vi "Periodic Tasks.vi"(8 "error in":errorcluster) -> ()   [LabVIEW 2019]
doc: "This VI runs in parallel to other tasks. It can contain as many user-defined periodic loops as you need. These can carry out PID or other sorts of timed response."
uses:
  Robot Global Data.vi
  <vilib>/Rock Robotics/WPI/ThirdParty/Phoenix-LabVIEW/Motor Controller/Controls/CTRE_Phoenix_MotorControl_ControlMode.ctl
  <vilib>/addons/control/pid/NI_PID_pid.lvlib
  <vilib>/Rock Robotics/Network Tables/NT Write Number.vi
  <vilib>/Rock Robotics/WPI/ThirdParty/Phoenix-LabVIEW/Motor Controller/Get/CTRE_Phoenix_MotorController_GetQuadratureData.vi
  <vilib>/addons/control/pid/pid.llb/PID (DBL).vi
  servoCameraStates.ctl
  <vilib>/Rock Robotics/WPI/ThirdParty/Phoenix-LabVIEW/Motor Controller/Controls/CTRE_Phoenix_MotorControl_LimitSwitchSource_Local.ctl
  <vilib>/Rock Robotics/WPI/ThirdParty/Phoenix-LabVIEW/Motor Controller/Controls/CTRE_Phoenix_MotorControl_LimitSwitchNormal.ctl
  <vilib>/Rock Robotics/WPI/ThirdParty/Phoenix-LabVIEW/Motor Controller/Get/CTRE_Phoenix_MotorController_GetLimitSwitchStates.vi
  <vilib>/Rock Robotics/Network Tables/NT Read Number.vi
panel:
  out "Waveform Chart":T1(graph)
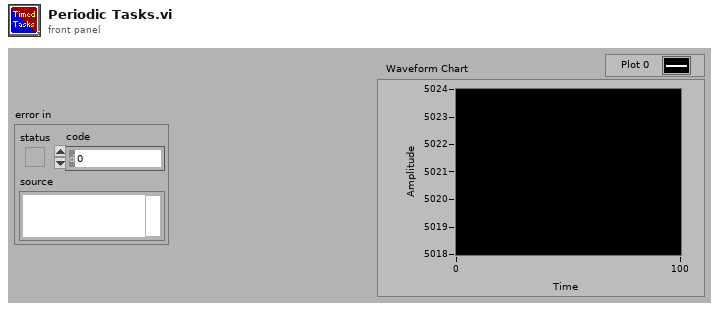
[diagram p1: front panel]
types:
  T1 = cluster{"intakePivotMotorActualAngle":dbl, "intakePivotMotorWantedAngle":dbl}
  T2 = typedef "CTRE_Phoenix_MotorControl_ControlMode.ctl" = u16
  T3 = typedef "WPI_MotorControlDeviceRef.ctl" = cluster{"DeviceStatus":errorcluster, "Type":T4, "PWM":cluster{"PWM Channel":T5, "DeadBand":T6}, "CAN":cluster{"Device Number":u8, "SetOutput VI Ref":variant, "GetOutput VI Ref":variant, "Enable VI Ref":variant, "Disable VI Ref":variant, "Data":variant}, "Invert":bool, "DIO PWM":cluster{"PWM \"Enable\" Channel":T5, "DIOChannel":T7, "PWM Rate":dbl}}
  T4 = typedef "WPI_MotorControlType.ctl" = enum16{"PWM", "CAN", "DIO PWM"}
  T5 = typedef "FPGA_DIOPWMChannel.ctl" = enum8{"PWM 0", "PWM 1", "PWM 2", "PWM 3", "PWM 4", "PWM 5", "PWM 6", "PWM 7", "PWM 8", "PWM 9", "PWM MXP 0", "PWM MXP 1", "PWM MXP 2", "PWM MXP 3", "PWM MXP 4", "PWM MXP 5", "PWM MXP 6", "PWM MXP 7", "PWM MXP 8", "PWM MXP 9", "Invalid"}
  T6 = typedef "WPI_PWMDeadband.ctl" = cluster{"Name":string, "maxPositivePwm":i32, "minPositivePwm":i32, "centerPwm":i32, "maxNegativePwm":i32, "minNegativePwm":i32, "angularRange":u16}
  T7 = typedef "FPGA_DIOChannel.ctl" = enum8{"DIO 0", "DIO 1", "DIO 2", "DIO 3", "DIO 4", "DIO 5", "DIO 6", "DIO 7", "DIO 8", "DIO 9", "DIO MXP 0", "DIO MXP 1", "DIO MXP 2", "DIO MXP 3", "DIO MXP 4", "DIO MXP 5", "DIO MXP 6", "DIO MXP 7", "DIO MXP 8", "DIO MXP 9", "DIO MXP 10", "DIO MXP 11", "DIO MXP 12", "DIO MXP 13", "DIO MXP 14", "DIO MXP 15", "SPI Port CS1", "SPI Port CS2", "SPI Port CS3", "SPI Port MISO", "SPI Port MOSI", "Invalid"}
  T8 = typedef "WPI_DriverStationRobotMode2.ctl" = enum16{"Autonomous Disabled", "Autonomous Enabled", "Teleop Disabled", "Teleop Enabled", "Disconnected", "Finish", "Test Disabled", "Test Enabled", "Emergency Stopped"}
  T9 = typedef "WPI_RobotDriveDevRef.ctl" = cluster{"DevStatus":errorcluster, "Motors[]":T3[], "Square Inputs":bool, "Max Output":dbl}
  T10 = cluster{"proportional gain (Kc)":dbl, "integral time (Ti, min)":dbl, "derivative time (Td, min)":dbl}
  T11 = typedef "CTRE_Phoenix_MotorControl_LimitSwitchNormal.ctl" = enum16{"Normally Open", "Normally Closed", "Disabled"}
  T12 = typedef "CTRE_Phoenix_MotorControl_LimitSwitchSource_Local.ctl" = enum16{"Feedback Connector", "Remote Talon SRX", "Remote CANifier", "Deactivated"}
  T13 = typedef "servoCameraStates.ctl" = enum16{"Up", "Out", "Down", ""}
  T14 = typedef "WPI_ServoDeviceRef.ctl" = cluster{"DeviceStatus":errorcluster, "PWM Channel":T5, "DeadBand":T6}
  T15 = typedef "WPI_CounterDevRef.ctl" = cluster{"DevStatus":errorcluster, "CntIndex":T16}
  T16 = typedef "FPGA_CounterCtrSystemIndex.ctl" = enum8{"Ctr 0", "Ctr 1", "Ctr 2", "Ctr 3", "Ctr 4", "Ctr 5", "Ctr 6", "Ctr 7", "Invalid"}
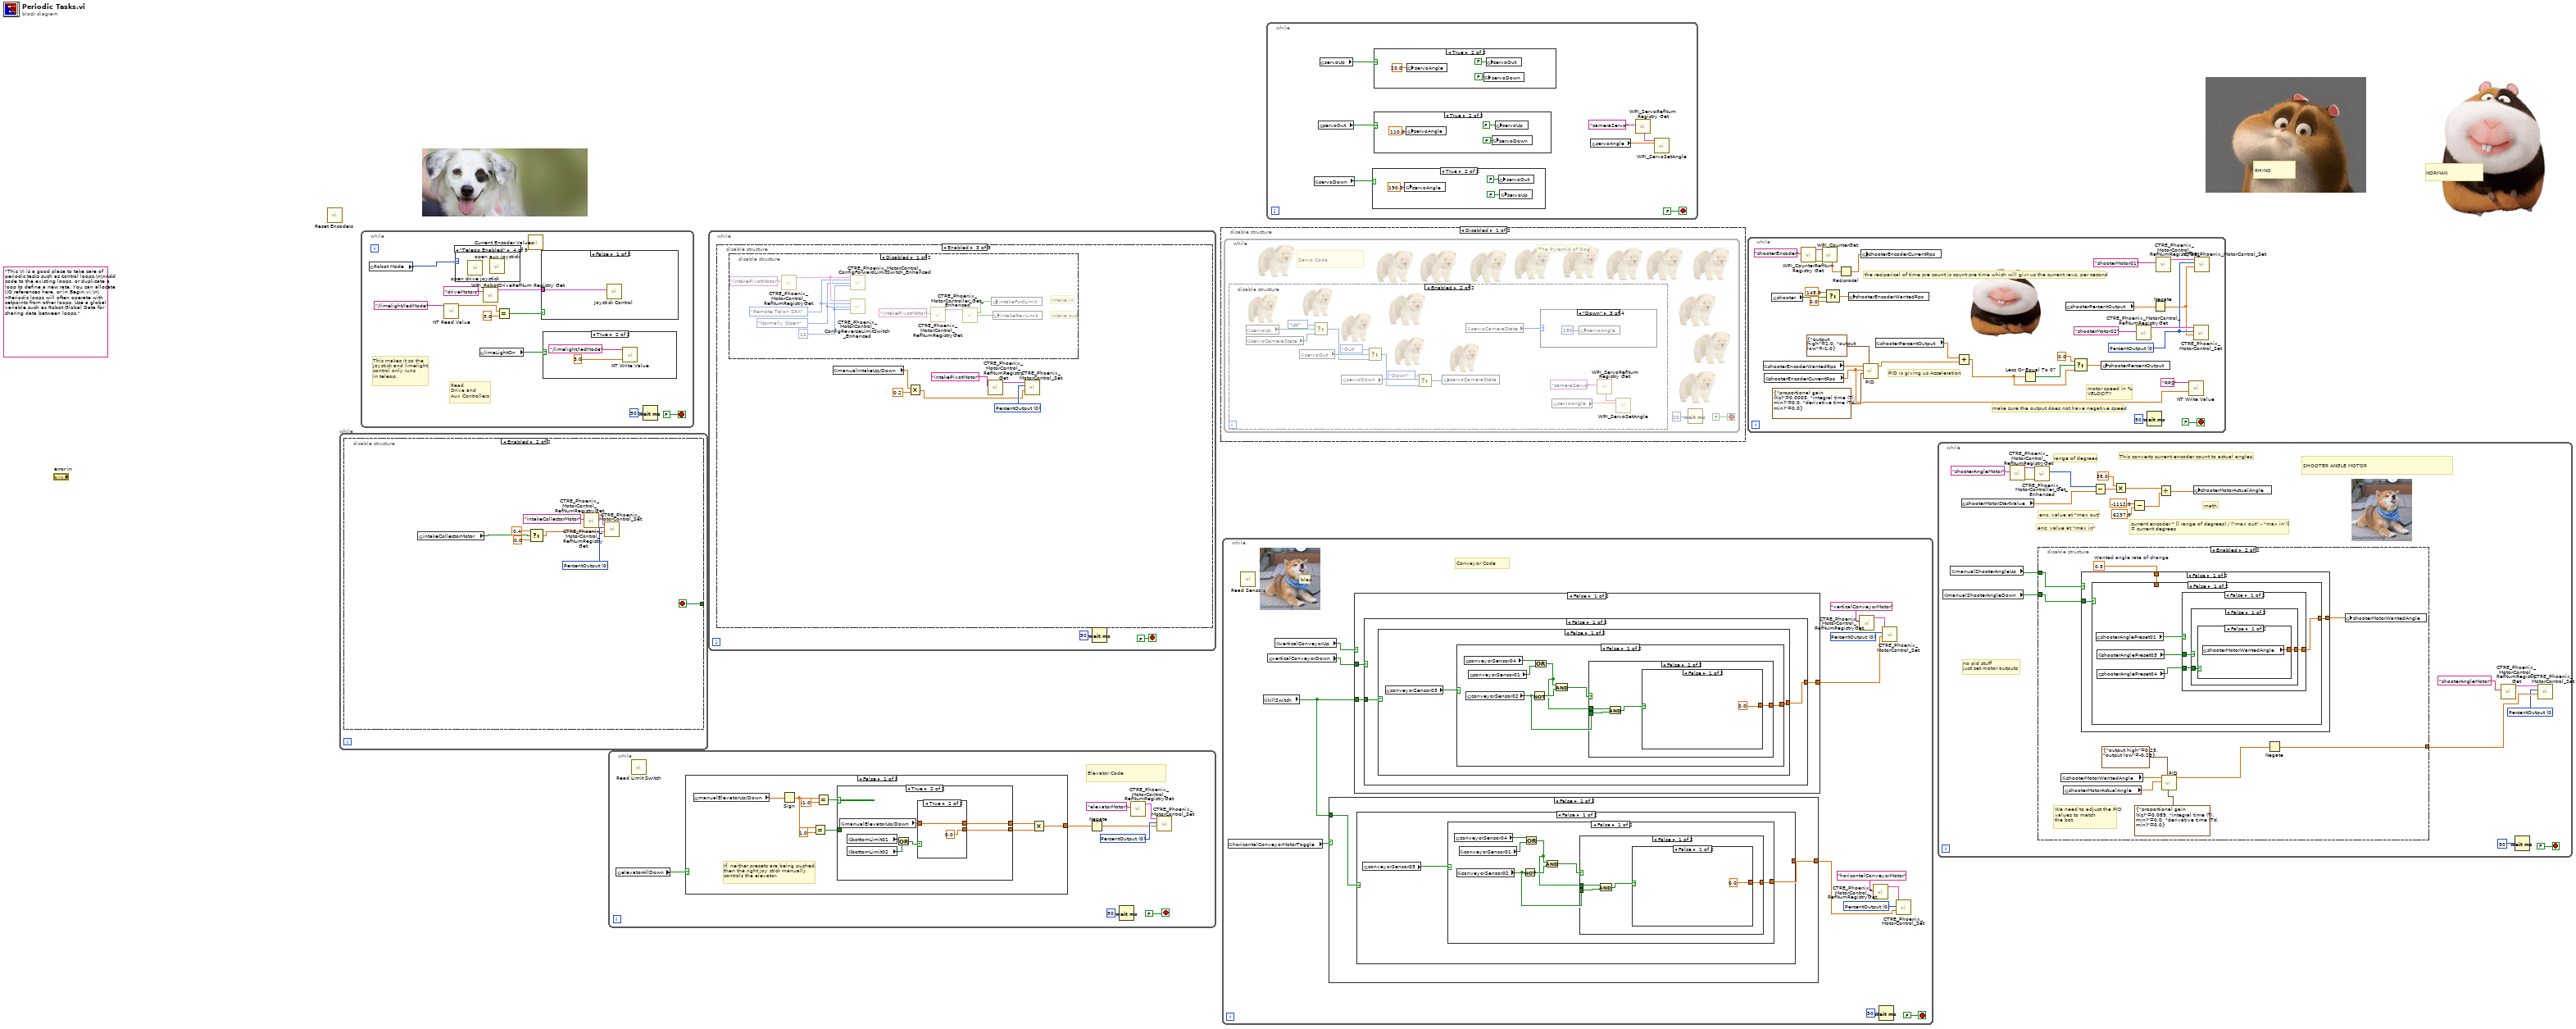
[diagram p0: block diagram]
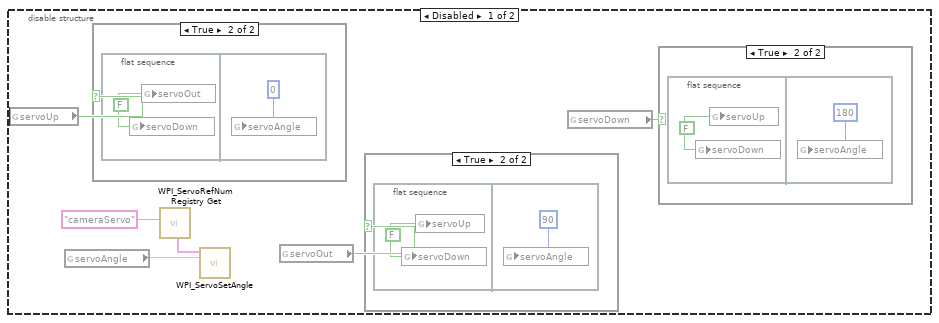
[diagram p5: hidden frame]
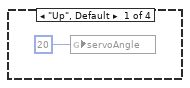
[diagram p9: hidden frame]
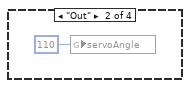
[diagram p10: hidden frame]
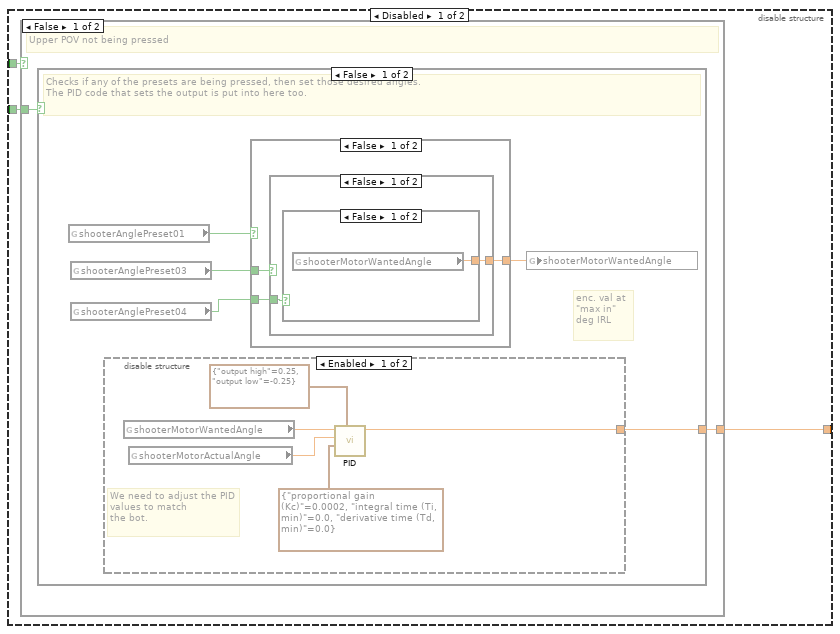
[diagram p13: hidden frame]
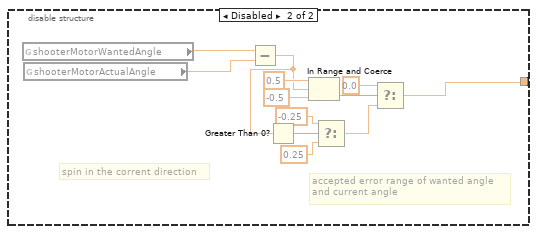
[diagram p14: hidden frame]
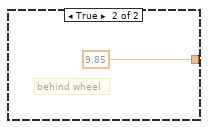
[diagram p15: hidden frame]
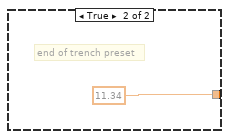
[diagram p16: hidden frame]
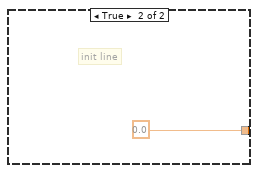
[diagram p17: hidden frame]
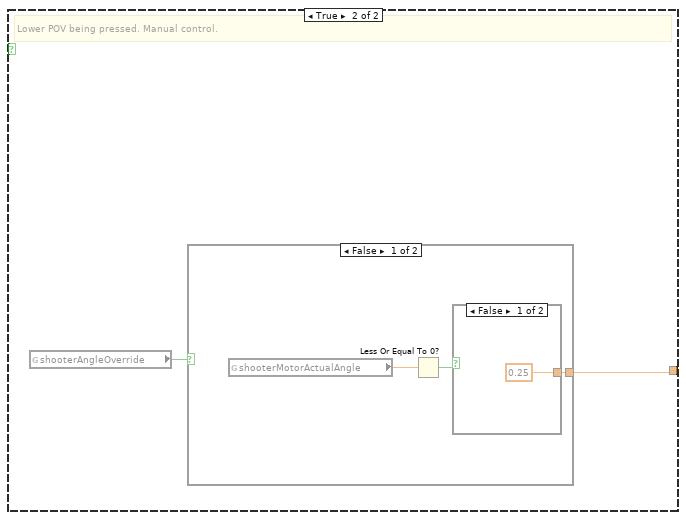
[diagram p18: hidden frame]
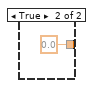
[diagram p19: hidden frame]
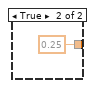
[diagram p20: hidden frame]
diagram:
  (unwired) "This VI is a good place to take care of periodic tasks such as control loops.\n\nAdd code to the existing loops, or duplicate a loop to define a new rate. You can allocate I/O references here, or in Begin.vi.\n\nPeriodic loops will often operate with setpoints from other loops. Use a global variable such as Robot Global Data for sharing data between loops."
  # "RHINO"
  # "NORMAN"
  n1 = call "Reset Encoders.vi"() -> ()  [unwired: 12 in]
  n2 = while {
    stop <- w1 stop-if-true
    n3 = disable-structure shown="Enabled" {
      disable-tunnel: [FALSE _] -> w1
      frame Disabled {
        w17 = T2 0 items=["PercentOutput"=0, "Position"=1, "Velocity"=2, "Current"=3, "Follower"=5, "MotionProfile"=6, "MotionMagic"=7, "MotionProfileArc"=10, "Disabled"=15] ("Control Mode")
        # "math"
        # "current encoder * [( range of degrees) / (\"max out\" - \"max in')]\n= current degrees"
        # "enc. value at \"max in\""
        # "enc. value at \"max out\""
        # "This converts current encoder count to actual angles."
        # "range of degrees"
        # "Check if motor value\nneeds to be negative\nor not."
        # "This chunk of code checks the current angle of the \nintake pivot motor. \nIf the motor is at or more of the desired \"all the way out\" \nangle then the intake collector motor begins to spin.\nIf the angle goes out of the range the motor will stop."
        # "All the way out intake angle."
        # "Intake Collector Code"
        n4 = global read "Robot Global Data.vi" "intakePivotMotorStartValue"() -> (w10:dbl)
        n5 = call <vilib>:"CTRE_Phoenix_MotorControl_RefNumRegistryGet.vi"("refnum name"="intakePivotMotor") -> ("error out"=w11:errorcluster, "PhoenixMotorControlDevRef"=w12:T3)  [unwired: 9 in]
        n6 = call-poly <vilib>:"CTRE_Phoenix_MotorController_Get_Enhanced.vi"("PhoenixMotorControlDevRef"=w12, "error in"=w11) -> ("Quadrature Position"=w2:i32)  [unwired: 10 in, 3 out]
        n7 = global read "Robot Global Data.vi" "intakePivotMotorActualAngle"() -> (w21:dbl)
        n8 = global write "Robot Global Data.vi" "intakePivotMotorActualValue"(w2) -> ()
        n9 = Subtract(x=w2, y=w10) -> (x-y=w9:dbl)
        n10 = Greater Or Equal?(x=w21, y=35.0 ("upper limit")) -> (x >= y?=w19:bool)
        n11 = Multiply(x=87.0, y=w9) -> (x*y=w5:dbl)
        n12 = case shown="True" w19 {
          tunnel: [0.0 0.4] -> w15
          frame False {
          }
          frame True {
          }
        }
        n13 = Subtract(x=-851.0, y=-20.0) -> (x-y=w4:dbl)
        n14 = Divide(x=w5, y=w4) -> (x/y=w3:dbl)
        n15 = global write "Robot Global Data.vi" "intakePivotMotorActualAngle"(w3) -> ()
        n16 = Wait (ms)(milliseconds to wait=u32 50) -> ()  [unwired: 1 out]
        n17 = call <vilib>:"CTRE_Phoenix_MotorControl_RefNumRegistryGet.vi"("refnum name"="intakeCollectorMotor") -> ("PhoenixMotorControlDevRef"=w18:T3)  [unwired: 9 in, 1 out]
        n18 = call <vilib>:"CTRE_Phoenix_MotorControl_Set.vi"("Output"=w15, "Control Mode"=w17, "PhoenixMotorControlDevRef"=w18) -> ()  [unwired: 7 in, 2 out]
      }
      frame Enabled {
        w30 = T2 0 items=["PercentOutput"=0, "Position"=1, "Velocity"=2, "Current"=3, "Follower"=5, "MotionProfile"=6, "MotionMagic"=7, "MotionProfileArc"=10, "Disabled"=15] ("Control Mode")
        (unwired) T2 0 items=["PercentOutput"=0, "Position"=1, "Velocity"=2, "Current"=3, "Follower"=5, "MotionProfile"=6, "MotionMagic"=7, "MotionProfileArc"=10, "Disabled"=15] ("Control Mode")
        n19 = global read "Robot Global Data.vi" "intakeCollectorMotor"() -> (w25:bool)
        n20 = Select(t=0.4, s=w25, f=0.0) -> (s? t:f=w28:dbl)
        n21 = call <vilib>:"CTRE_Phoenix_MotorControl_RefNumRegistryGet.vi"("refnum name"="intakeCollectorMotor") -> ("PhoenixMotorControlDevRef"=w31:T3)  [unwired: 9 in, 1 out]
        n22 = call <vilib>:"CTRE_Phoenix_MotorControl_RefNumRegistryGet.vi"("refnum name"="intakeCollectorMotor") -> ()  [unwired: 9 in, 2 out]
        n23 = call <vilib>:"CTRE_Phoenix_MotorControl_Set.vi"("Output"=w28, "Control Mode"=w30, "PhoenixMotorControlDevRef"=w31) -> ()  [unwired: 7 in, 2 out]
      }
    }
  }
  n24 = while {
    stop <- FALSE stop-if-true
    # "Read\nDrive and\nAux Controllers"
    # "This makes it so the\njoystick and limelight\ncontrol only runs\nin teleop."
    n25 = global read "Robot Global Data.vi" "Robot Mode"() -> (w33:T8)
    n26 = call-poly <vilib>:"NT Read Value.vi"("Name"="/limelight/ledMode") -> ("Numeric"=w35:dbl)  [unwired: 9 in, 1 out]
    n27 = case shown="\"Teleop Enabled\"" w33 {
      frame "Autonomous Disabled", Default {
        n28 = call "open drive joystick.vi"() -> ()  [unwired: 12 in]
        n29 = call "open aux joystick.vi"() -> ()  [unwired: 12 in]
      }
      frame "Autonomous Enabled" {
      }
      frame "Teleop Disabled" {
        n30 = call "open drive joystick.vi"() -> ()  [unwired: 12 in]
        n31 = call "open aux joystick.vi"() -> ()  [unwired: 12 in]
      }
      frame "Teleop Enabled" {
        n32 = call "open drive joystick.vi"() -> ()  [unwired: 12 in]
        n33 = call "open aux joystick.vi"() -> ()  [unwired: 12 in]
      }
      frame "Disconnected" {
        n34 = call "open drive joystick.vi"() -> ()  [unwired: 12 in]
        n35 = call "open aux joystick.vi"() -> ()  [unwired: 12 in]
      }
      frame "Finish" {
        n36 = call "open drive joystick.vi"() -> ()  [unwired: 12 in]
        n37 = call "open aux joystick.vi"() -> ()  [unwired: 12 in]
      }
      frame "Test Disabled" {
        n38 = call "open drive joystick.vi"() -> ()  [unwired: 12 in]
        n39 = call "open aux joystick.vi"() -> ()  [unwired: 12 in]
      }
      frame "Test Enabled" {
        n40 = call "open drive joystick.vi"() -> ()  [unwired: 12 in]
        n41 = call "open aux joystick.vi"() -> ()  [unwired: 12 in]
      }
      frame "Emergency Stopped" {
        n42 = call "open drive joystick.vi"() -> ()  [unwired: 12 in]
        n43 = call "open aux joystick.vi"() -> ()  [unwired: 12 in]
      }
    }
    n44 = global read "Robot Global Data.vi" "limeLightOn"() -> (w38:bool)
    n45 = call <vilib>:"WPI_RobotDriveRefNum Registry Get.vi"("refnum name"="driveMotors") -> ("RobotDriveDevRef"=w39:T9)  [unwired: 9 in, 1 out]
    n46 = Equal?(x=w35, y=3.0) -> (x = y?=w34:bool)
    n47 = call "Current Encoder Values.vi"() -> ()  [unwired: 12 in]
    n48 = case shown="False" w34 {
      tunnel: w39 -> [w47 w48]
      frame False {
        n49 = call "Joystick Control.vi"("RobotDriveDevRef"=w47) -> ()  [unwired: 11 in]
      }
      frame True {
        # "sounds cool"
        n50 = call "Limelight Control.vi"("input cluster"=w48) -> ()  [unwired: 11 in]
      }
    }
    n51 = case shown="True" w38 {
      frame False {
        n52 = call-poly <vilib>:"NT Write Value.vi"("Numeric"=1.0, "Name"="/limelight/ledMode") -> ()  [unwired: 9 in, 1 out]
      }
      frame True {
        n53 = call-poly <vilib>:"NT Write Value.vi"("Numeric"=3.0, "Name"="/limelight/ledMode") -> ()  [unwired: 9 in, 1 out]
      }
    }
    n54 = Wait (ms)(milliseconds to wait=u32 50) -> ()  [unwired: 1 out]
  }
  n55 = while {
    stop <- FALSE stop-if-true
    w53 = T2 0 items=["PercentOutput"=0, "Position"=1, "Velocity"=2, "Current"=3, "Follower"=5, "MotionProfile"=6, "MotionMagic"=7, "MotionProfileArc"=10, "Disabled"=15] ("Control Mode")
    # "Elevator Code"
    n56 = global read "Robot Global Data.vi" "elevatorAllDown"() -> (w50:bool)
    n57 = call "Read Limit Switch.vi"() -> ()  [unwired: 12 in]
    n58 = case shown="False" w50 {
      tunnel: [w65 w94] -> w51
      frame False {
        # "If, neither presets are being pushed, \nthen the right joy stick manually \ncontrols the elevator."
        n59 = global read "Robot Global Data.vi" "manualElevatorUp/Down"() -> (w64:dbl)
        n60 = Sign(1:w64) -> (0:w59:dbl)
        n61 = Equal?(x=w59, y=1.0) -> (x = y?=w57:bool)
        n62 = Equal?(x=w59, y=-1.0) -> (x = y?=w63:bool)
        n63 = case shown="True" w63 {
          tunnel: [w66 w83] -> w61
          tunnel: [w67 w81] -> w60
          tunnel: w57 -> [w68 _]
          frame False {
            n64 = case shown="False" w68 {
              tunnel: [0.0 w73] -> w67
              tunnel: [0.0 w72] -> w66
              frame False {
              }
              frame True {
                n65 = global read "Robot Global Data.vi" "manualElevatorUp/Down"() -> (w74:dbl)
                n66 = global read "Robot Global Data.vi" "upperLimit01"() -> (w75:bool)
                n67 = global read "Robot Global Data.vi" "upperLimit02"() -> (w76:bool)
                n68 = Or(x=w75, y=w76) -> (x .or. y?=w71:bool)
                n69 = case shown="False" w71 {
                  tunnel: w74 -> [w77 w80]
                  tunnel: [w77 w80] -> w73
                  tunnel: [1.0 0.0] -> w72
                  frame False {
                  }
                  frame True {
                  }
                }
              }
            }
          }
          frame True {
            n70 = global read "Robot Global Data.vi" "manualElevatorUp/Down"() -> (w82:dbl)
            n71 = global read "Robot Global Data.vi" "bottomLimit01"() -> (w85:bool)
            n72 = global read "Robot Global Data.vi" "bottomLimit02"() -> (w86:bool)
            n73 = Or(x=w85, y=w86) -> (x .or. y?=w84:bool)
            n74 = case shown="True" w84 {
              tunnel: [1.0 0.0] -> w83
              tunnel: w82 -> [w88 w89]
              tunnel: [w88 w89] -> w81
              frame False {
              }
              frame True {
              }
            }
          }
        }
        n75 = Multiply(x=w60, y=w61) -> (x*y=w65:dbl)
      }
      frame True {
        # "the elevator will keep moving down\nuntil the lower limit switch turns true."
        n76 = global read "Robot Global Data.vi" "bottomLimit01"() -> (w91:bool)
        n77 = global read "Robot Global Data.vi" "bottomLimit02"() -> (w92:bool)
        n78 = Or(x=w91, y=w92) -> (x .or. y?=w93:bool)
        n79 = case shown="False" w93 {
          tunnel: [w95 0.0] -> w94
          frame False {
            n80 = Negate(x=0.8) -> (-x=w95:dbl)
          }
          frame True {
          }
        }
      }
    }
    n81 = Negate(x=w51) -> (-x=w49:dbl)
    n82 = Wait (ms)(milliseconds to wait=u32 50) -> ()  [unwired: 1 out]
    n83 = call <vilib>:"CTRE_Phoenix_MotorControl_RefNumRegistryGet.vi"("refnum name"="elevatorMotor") -> ("PhoenixMotorControlDevRef"=w52:T3)  [unwired: 9 in, 1 out]
    n84 = call <vilib>:"CTRE_Phoenix_MotorControl_Set.vi"("Output"=w49, "Control Mode"=w53, "PhoenixMotorControlDevRef"=w52) -> ()  [unwired: 7 in, 2 out]
  }
  n85 = while {
    stop <- FALSE stop-if-true
    n86 = disable-structure shown="Enabled" {
      frame Disabled {
        w116 = T2 0 items=["PercentOutput"=0, "Position"=1, "Velocity"=2, "Current"=3, "Follower"=5, "MotionProfile"=6, "MotionMagic"=7, "MotionProfileArc"=10, "Disabled"=15] ("Control Mode")
        # "This chunk of code actually gives the\nintake pivot motor a value by comparing\nthe actual to the wanted and then doing \nmath."
        # "This chunk of code see's if either preset\nbutton is being pressed, then gives the\ndesired angle depending on which button\nis being pressed. If neither button is being\npressed, then the left joystick on the aux\ncontrols the pivot motor."
        # "We need to adjust the PID values to match \nthe bot."
        # "We need to get the preset\nangles for the intake as \nsoon as we get the robot."
        # "Use this to scale the rate at which the\nwanted angle changes based on the joystick"
        n87 = global read "Robot Global Data.vi" "intakePivotMotorWantedAngle"() -> (w103:dbl)
        n88 = global read "Robot Global Data.vi" "intakePivotMotorActualAngle"() -> (w104:dbl)
        n89 = global read "Robot Global Data.vi" "manualIntakeUp/Down"() -> (w125:dbl)
        n90 = global read "Robot Global Data.vi" "intakeOut"() -> (w124:bool)
        n91 = global read "Robot Global Data.vi" "intakeIn"() -> (w122)
        n92 = Or(x=w122, y=w124) -> (x .or. y?=w123:bool)
        n93 = call <vilib>:"CTRE_Phoenix_MotorControl_RefNumRegistryGet.vi"("refnum name"="intakePivotMotor") -> ("error out"=w113:errorcluster, "PhoenixMotorControlDevRef"=w114:T3)  [unwired: 9 in]
        n94 = Multiply(x=1.0, y=w125) -> (x*y=w120:dbl)
        n95 = call-poly <vilib>:"CTRE_Phoenix_MotorController_Get_Enhanced.vi"("PhoenixMotorControlDevRef"=w114, "error in"=w113) -> ("Quadrature Position"=w111:i32)  [unwired: 10 in, 3 out]
        n96 = call-poly <vilib>:"PID.vi"("output range"=cluster{"output high":dbl, "output low":dbl} {"output high"=0.2, "output low"=-0.2}, "PID gains"=T10 {"proportional gain (Kc)"=0.015, "integral time (Ti, min)"=0.0, "derivative time (Td, min)"=0.0}, "process variable"=w103, "setpoint"=w104) -> ("output"=w101:dbl)  [unwired: 6 in, 1 out]
        n97 = case shown="False" w123 {
          tunnel: w122 -> [_ w131]
          tunnel: [w127 w130] -> w121
          tunnel: w120 -> [w128 _]
          frame False {
            # "Neither Preset buttons \nare being pressed.\n\nThis allows the Left Y\njoystick to control the \nActual Angle"
            n98 = global read "Robot Global Data.vi" "intakePivotMotorWantedAngle"() -> (w129:dbl)
            n99 = Add(x=w129, y=w128) -> (x+y=w127:dbl)
          }
          frame True {
            n100 = case shown="False" w131 {
              tunnel: [5018.0 5192.0] -> w130
              frame False {
                # "Preset angle for \nintake at Out Position"
              }
              frame True {
                # "Preset Angle for\nIntake at Vertical \nPosition"
              }
            }
          }
        }
        n101 = Negate(x=w101) -> (-x=w100:dbl)
        n102 = Subtract(x=960.0, y=24.0) -> (x-y=w107:dbl)
        n103 = Bundle("intakePivotMotorActualAngle"=w104, "intakePivotMotorWantedAngle"=w103) -> (→"Waveform Chart":T1)  [unwired: 1 in]
        n104 = call <vilib>:"CTRE_Phoenix_MotorControl_RefNumRegistryGet.vi"("refnum name"="intakePivotMotor") -> ("PhoenixMotorControlDevRef"=w117:T3)  [unwired: 9 in, 1 out]
        n105 = Divide(x=180.0, y=w107) -> (x/y=w106:dbl)
        n106 = call <vilib>:"CTRE_Phoenix_MotorControl_Set.vi"("Output"=w100, "Control Mode"=w116, "PhoenixMotorControlDevRef"=w117) -> ()  [unwired: 7 in, 2 out]
        n107 = Multiply(x=w106, y=w111) -> (x*y=w112:dbl)
        n108 = global write "Robot Global Data.vi" "intakePivotMotorActualAngle"(w112) -> ()
        n109 = global write "Robot Global Data.vi" "intakePivotMotorWantedAngle"(w121) -> ()
      }
      frame Disabled {
        w149 = T2 0 items=["PercentOutput"=0, "Position"=1, "Velocity"=2, "Current"=3, "Follower"=5, "MotionProfile"=6, "MotionMagic"=7, "MotionProfileArc"=10, "Disabled"=15] ("Control Mode")
        # "INTAKE PIVOT MOTOR CODE"
        # "math"
        # "current encoder * [( range of degrees) / (\"max out\" - \"max in')]\n= current degrees"
        # "enc. value at \"max in\""
        # "enc. value at \"max out\""
        # "This converts current encoder count to actual angles."
        # "range of degrees"
        n110 = global read "Robot Global Data.vi" "intakePivotMotorStartValue"() -> (w142:dbl)
        n111 = call <vilib>:"CTRE_Phoenix_MotorControl_RefNumRegistryGet.vi"("refnum name"="intakePivotMotor") -> ("error out"=w143:errorcluster, "PhoenixMotorControlDevRef"=w144:T3)  [unwired: 9 in]
        n112 = global read "Robot Global Data.vi" "manualIntakeUp/Down"() -> (w148:dbl)
        n113 = call-poly <vilib>:"CTRE_Phoenix_MotorController_Get_Enhanced.vi"("PhoenixMotorControlDevRef"=w144, "error in"=w143) -> ("Quadrature Position"=w134:i32)  [unwired: 10 in, 3 out]
        n114 = global write "Robot Global Data.vi" "intakePivotMotorActualValue"(w134) -> ()
        n115 = Multiply(x=w148, y=0.2) -> (x*y=w146:dbl)
        n116 = Subtract(x=w134, y=w142) -> (x-y=w141:dbl)
        n117 = Multiply(x=87.0, y=w141) -> (x*y=w137:dbl)
        n118 = Subtract(x=-851.0, y=-20.0) -> (x-y=w136:dbl)
        n119 = call <vilib>:"CTRE_Phoenix_MotorControl_RefNumRegistryGet.vi"("refnum name"="intakePivotMotor") -> ("PhoenixMotorControlDevRef"=w150:T3)  [unwired: 9 in, 1 out]
        n120 = Divide(x=w137, y=w136) -> (x/y=w135:dbl)
        n121 = call <vilib>:"CTRE_Phoenix_MotorControl_Set.vi"("Output"=w146, "Control Mode"=w149, "PhoenixMotorControlDevRef"=w150) -> ()  [unwired: 7 in, 2 out]
        n122 = global write "Robot Global Data.vi" "intakePivotMotorActualAngle"(w135) -> ()
      }
      frame Enabled {
        w155 = T2 0 items=["PercentOutput"=0, "Position"=1, "Velocity"=2, "Current"=3, "Follower"=5, "MotionProfile"=6, "MotionMagic"=7, "MotionProfileArc"=10, "Disabled"=15] ("Control Mode")
        n123 = disable-structure shown="Disabled" {
          frame Disabled {
            w164 = 10 ("deviceID")
            w163 = CTRE_Phoenix_MotorControl_LimitSwitchNormal."Normally Open" ("NormallyOpenOrClosed")
            w162 = CTRE_Phoenix_MotorControl_LimitSwitchSource_Local."Remote Talon SRX" ("Limit Switch Source")
            # "intake out"
            # "intake in"
            n124 = call <vilib>:"CTRE_Phoenix_MotorControl_RefNumRegistryGet.vi"("refnum name"="intakePivotMotor") -> ("PhoenixMotorControlDevRef"=w165:T3)  [unwired: 9 in, 1 out]
            n125 = call <vilib>:"CTRE_Phoenix_MotorControl_ConfigForwardLimitSwitch_Enhanced.vi"("PhoenixMotorControlDevRef"=w165, "Limit Switch Source"=w162, "NormallyOpenOrClosed"=w163, "deviceID"=w164) -> ()  [unwired: 10 in, 2 out]
            n126 = call <vilib>:"CTRE_Phoenix_MotorControl_ConfigReverseLimitSwitch_Enhanced.vi"("PhoenixMotorControlDevRef"=w165, "Limit Switch Source"=w162, "NormallyOpenOrClosed"=w163, "deviceID"=w164) -> ()  [unwired: 10 in, 2 out]
            n127 = call <vilib>:"CTRE_Phoenix_MotorControl_RefNumRegistryGet.vi"("refnum name"="intakePivotMotor") -> ("PhoenixMotorControlDevRef"=w161:T3)  [unwired: 9 in, 1 out]
            n128 = call-poly <vilib>:"CTRE_Phoenix_MotorController_Get_Enhanced.vi"("PhoenixMotorControlDevRef"=w161) -> ("Forward Limit Closed?"=w158:bool, "Reverse Limit Closed?"=w159:bool)  [unwired: 11 in, 2 out]
            n129 = global write "Robot Global Data.vi" "intakeFwdLimit"(w158) -> ()
            n130 = global write "Robot Global Data.vi" "intakeRevLimit"(w159) -> ()
          }
          frame Enabled {
          }
        }
        n131 = global read "Robot Global Data.vi" "manualIntakeUp/Down"() -> (w154:dbl)
        n132 = Multiply(x=w154, y=0.2) -> (x*y=w152:dbl)
        n133 = call <vilib>:"CTRE_Phoenix_MotorControl_RefNumRegistryGet.vi"("refnum name"="intakePivotMotor") -> ("PhoenixMotorControlDevRef"=w156:T3)  [unwired: 9 in, 1 out]
        n134 = call <vilib>:"CTRE_Phoenix_MotorControl_Set.vi"("Output"=w152, "Control Mode"=w155, "PhoenixMotorControlDevRef"=w156) -> ()  [unwired: 7 in, 2 out]
      }
      frame Disabled {
        w169 = T2 0 items=["PercentOutput"=0, "Position"=1, "Velocity"=2, "Current"=3, "Follower"=5, "MotionProfile"=6, "MotionMagic"=7, "MotionProfileArc"=10, "Disabled"=15] ("Control Mode")
        n135 = global read "Robot Global Data.vi" "manualIntakeUp/Down"() -> (w167:dbl)
        n136 = global read "Robot Global Data.vi" "intakeOut"() -> (w176:bool)
        n137 = global read "Robot Global Data.vi" "intakeIn"() -> (w178)
        n138 = Or(x=w178, y=w176) -> (x .or. y?=w177:bool)
        n139 = call <vilib>:"CTRE_Phoenix_MotorControl_RefNumRegistryGet.vi"("refnum name"="intakePivotMotor") -> ("error out"=w180:errorcluster, "PhoenixMotorControlDevRef"=w179:T3)  [unwired: 9 in]
        n140 = call-poly <vilib>:"CTRE_Phoenix_MotorController_Get_Enhanced.vi"("PhoenixMotorControlDevRef"=w179, "error in"=w180) -> ("Quadrature Position"=w182:i32)  [unwired: 10 in, 3 out]
        n141 = case shown="False" w177 {
          tunnel: w178 -> [_ w189]
          tunnel: [w185 w188] -> w168
          tunnel: w167 -> [w186 _]
          frame False {
            # "Neither Preset buttons \nare being pressed.\n\nThis allows the Left Y\njoystick to control the \nActual Angle"
            n142 = Multiply(x=w186, y=0.2) -> (x*y=w185:dbl)
          }
          frame True {
            n143 = case shown="True" w189 {
              tunnel: [w193 w199] -> w188
              frame False {
                n144 = global read "Robot Global Data.vi" "intakePivotMotorActualAngle"() -> (w192:dbl)
                n145 = Less Or Equal?(x=w192, y=5018.0) -> (x <= y?=w190:bool)
                n146 = Select(t=0.0, s=w190, f=-0.2) -> (s? t:f=w193:dbl)
              }
              frame True {
                n147 = global read "Robot Global Data.vi" "intakePivotMotorActualAngle"() -> (w198:dbl)
                n148 = Greater Or Equal?(x=w198, y=5192.0) -> (x >= y?=w196:bool)
                n149 = Select(t=0.0, s=w196, f=0.2) -> (s? t:f=w199:dbl)
              }
            }
          }
        }
        n150 = Subtract(x=960.0, y=24.0) -> (x-y=w183:dbl)
        n151 = Divide(x=180.0, y=w183) -> (x/y=w184:dbl)
        n152 = Multiply(x=w184, y=w182) -> (x*y=w181:dbl)
        n153 = global write "Robot Global Data.vi" "intakePivotMotorActualAngle"(w181) -> ()
        n154 = call <vilib>:"CTRE_Phoenix_MotorControl_RefNumRegistryGet.vi"("refnum name"="intakePivotMotor") -> ("PhoenixMotorControlDevRef"=w170:T3)  [unwired: 9 in, 1 out]
        n155 = call <vilib>:"CTRE_Phoenix_MotorControl_Set.vi"("Output"=w168, "Control Mode"=w169, "PhoenixMotorControlDevRef"=w170) -> ()  [unwired: 7 in, 2 out]
      }
      frame Disabled {
        w218 = T2 0 items=["PercentOutput"=0, "Position"=1, "Velocity"=2, "Current"=3, "Follower"=5, "MotionProfile"=6, "MotionMagic"=7, "MotionProfileArc"=10, "Disabled"=15] ("Control Mode")
        # "0.017"
        # "prevent manuall adjustment from going out of\nacceptable angels. alos give the drivers the option to push\nfutther than the angel presets by 5 degrees."
        # "INTAKE PIVOT MOTOR CODE"
        # "We need to adjust the PID values to match \nthe bot."
        # "math"
        # "current encoder * [( range of degrees) / (\"max out\" - \"max in')]\n= current degrees"
        # "enc. value at \"max in\""
        # "enc. value at \"max out\""
        # "This converts current encoder count to actual angles."
        # "range of degrees"
        n156 = global read "Robot Global Data.vi" "manualIntakeUp/Down"() -> (w210:dbl)
        n157 = global read "Robot Global Data.vi" "intakePivotMotorStartValue"() -> (w232:dbl)
        n158 = global read "Robot Global Data.vi" "intakeOut"() -> (w216:bool)
        n159 = global read "Robot Global Data.vi" "intakeEat"() -> (w217:bool)
        n160 = global read "Robot Global Data.vi" "intakePivotMotorWantedAngle"() -> (w222:dbl)
        n161 = global read "Robot Global Data.vi" "intakePivotMotorActualAngle"() -> (w206:dbl)
        n162 = call <vilib>:"CTRE_Phoenix_MotorControl_RefNumRegistryGet.vi"("refnum name"="intakePivotMotor") -> ("error out"=w233:errorcluster, "PhoenixMotorControlDevRef"=w234:T3)  [unwired: 9 in]
        n163 = Negate(x=w210) -> (-x=w209:dbl)
        n164 = case shown="False" w217 {
          tunnel: w216 -> [w238 _]
          tunnel: [w237 -5.0] -> w214
          tunnel: w209 -> [w236 _]
          frame False {
            n165 = case shown="True" w238 {
              tunnel: [w239 85.0] -> w237
              tunnel: w236 -> [w242 _]
              frame False {
                # "Use this to scale the rate at which the\nwanted angle changes based on the joystick"
                n166 = global read "Robot Global Data.vi" "intakePivotMotorWantedAngle"() -> (w243:dbl)
                n167 = Multiply(x=w242, y=3.0) -> (x*y=w240:dbl)
                n168 = Add(x=w243, y=w240) -> (x+y=w239:dbl)
              }
              frame True {
              }
            }
          }
          frame True {
          }
        }
        n169 = call-poly <vilib>:"CTRE_Phoenix_MotorController_Get_Enhanced.vi"("PhoenixMotorControlDevRef"=w234, "error in"=w233) -> ("Quadrature Position"=w224:i32)  [unwired: 10 in, 3 out]
        n170 = global write "Robot Global Data.vi" "intakePivotMotorActualValue"(w224) -> ()
        n171 = call-poly <vilib>:"PID.vi"("output range"=cluster{"output high":dbl, "output low":dbl} {"output high"=0.2, "output low"=-0.2}, "PID gains"=T10 {"proportional gain (Kc)"=0.017, "integral time (Ti, min)"=0.0, "derivative time (Td, min)"=0.0}, "process variable"=w206, "setpoint"=w222) -> ("output"=w207:dbl)  [unwired: 6 in, 1 out]
        n172 = Subtract(x=w224, y=w232) -> (x-y=w231:dbl)
        n173 = Multiply(x=87.0, y=w231) -> (x*y=w227:dbl)
        n174 = Less Or Equal?(x=w206, y=45.0 ("x")) -> (x <= y?=w204:bool)
        n175 = Subtract(x=-851.0, y=-20.0) -> (x-y=w226:dbl)
        n176 = Add(x=0.015, y=w207) -> (x+y=w205:dbl)
        n177 = Select(t=w205, s=w204, f=w206) -> (s? t:f=w208:dbl)
        n178 = Divide(x=w227, y=w226) -> (x/y=w225:dbl)
        n179 = Negate(x=w208) -> (-x=w215:dbl)
        n180 = global write "Robot Global Data.vi" "intakePivotMotorActualAngle"(w225) -> ()
        n181 = call <vilib>:"CTRE_Phoenix_MotorControl_RefNumRegistryGet.vi"("refnum name"="intakePivotMotor") -> ("PhoenixMotorControlDevRef"=w219:T3)  [unwired: 9 in, 1 out]
        n182 = call <vilib>:"CTRE_Phoenix_MotorControl_Set.vi"("Output"=w215, "Control Mode"=w218, "PhoenixMotorControlDevRef"=w219) -> ()  [unwired: 7 in, 2 out]
        n183 = In Range and Coerce(upper limit=96.0 ("x"), x=w214, lower limit=-5.0) -> (coerced(x)=w213:dbl)  [unwired: 1 out]
        n184 = global write "Robot Global Data.vi" "intakePivotMotorWantedAngle"(w213) -> ()
      }
    }
    n185 = Wait (ms)(milliseconds to wait=u32 50) -> ()  [unwired: 1 out]
  }
  n186 = disable-structure shown="Disabled" {
    frame Disabled {
      n187 = while {
        stop <- FALSE stop-if-true
        # "The Pyramid of Dog"
        # "Servo Code"
        n188 = disable-structure shown="Enabled" {
          frame Disabled {
            n189 = global read "Robot Global Data.vi" "servoUp"() -> (w251:bool)
            n190 = global read "Robot Global Data.vi" "servoAngle"() -> (w250:dbl)
            n191 = case shown="True" w251 {
              frame False {
              }
              frame True {
                n192 = flat-sequence {
                  frame #0 {
                    w254 = FALSE
                    n193 = global write "Robot Global Data.vi" "servoDown"(w254) -> ()
                    n194 = global write "Robot Global Data.vi" "servoOut"(w254) -> ()
                  }
                  frame #1 {
                    n195 = global write "Robot Global Data.vi" "servoAngle"(0) -> ()
                  }
                }
              }
            }
            n196 = call <vilib>:"WPI_ServoRefNum Registry Get.vi"("refnum name"="cameraServo") -> ("ServoDeviceRef"=w253:T14)  [unwired: 9 in, 1 out]
            n197 = call <vilib>:"WPI_ServoSetAngle.vi"("Angle"=w250, "ServoDeviceRef"=w253) -> ()  [unwired: 8 in, 2 out]
            n198 = global read "Robot Global Data.vi" "servoOut"() -> (w248:bool)
            n199 = case shown="True" w248 {
              frame False {
              }
              frame True {
                n200 = flat-sequence {
                  frame #0 {
                    w256 = FALSE
                    n201 = global write "Robot Global Data.vi" "servoDown"(w256) -> ()
                    n202 = global write "Robot Global Data.vi" "servoUp"(w256) -> ()
                  }
                  frame #1 {
                    n203 = global write "Robot Global Data.vi" "servoAngle"(90) -> ()
                  }
                }
              }
            }
            n204 = global read "Robot Global Data.vi" "servoDown"() -> (w249:bool)
            n205 = case shown="True" w249 {
              frame False {
              }
              frame True {
                n206 = flat-sequence {
                  frame #0 {
                    w258 = FALSE
                    n207 = global write "Robot Global Data.vi" "servoDown"(w258) -> ()
                    n208 = global write "Robot Global Data.vi" "servoUp"(w258) -> ()
                  }
                  frame #1 {
                    n209 = global write "Robot Global Data.vi" "servoAngle"(180) -> ()
                  }
                }
              }
            }
          }
          frame Enabled {
            n210 = global read "Robot Global Data.vi" "servoUp"() -> (w273:bool)
            n211 = global read "Robot Global Data.vi" "servoCameraState"() -> (w264:T13)
            n212 = global read "Robot Global Data.vi" "servoOut"() -> (w271:bool)
            n213 = Select(t=servoCameraStates."Up" ("servoCameraState"), s=w273, f=w264) -> (s? t:f=w267:T13)
            n214 = global read "Robot Global Data.vi" "servoDown"() -> (w269:bool)
            n215 = Select(t=servoCameraStates."Out" ("servoCameraState"), s=w271, f=w267) -> (s? t:f=w266:T13)
            n216 = Select(t=servoCameraStates."Down" ("servoCameraState"), s=w269, f=w266) -> (s? t:f=w265:T13)
            n217 = global write "Robot Global Data.vi" "servoCameraState"(w265) -> ()
            n218 = global read "Robot Global Data.vi" "servoCameraState"() -> (w263:T13)
            n219 = case shown="\"Down\"" w263 {
              frame "Up", Default {
                n220 = global write "Robot Global Data.vi" "servoAngle"(20) -> ()
              }
              frame "Out" {
                n221 = global write "Robot Global Data.vi" "servoAngle"(110) -> ()
              }
              frame "Down" {
                n222 = global write "Robot Global Data.vi" "servoAngle"(190) -> ()
              }
              frame "" {
              }
            }
            n223 = global read "Robot Global Data.vi" "servoAngle"() -> (w260:dbl)
            n224 = call <vilib>:"WPI_ServoRefNum Registry Get.vi"("refnum name"="cameraServo") -> ("ServoDeviceRef"=w262:T14)  [unwired: 9 in, 1 out]
            n225 = call <vilib>:"WPI_ServoSetAngle.vi"("Angle"=w260, "ServoDeviceRef"=w262) -> ()  [unwired: 8 in, 2 out]
          }
        }
        n226 = Wait (ms)(milliseconds to wait=u32 20) -> ()  [unwired: 1 out]
      }
    }
    frame Enabled {
    }
  }
  n227 = while {
    stop <- FALSE stop-if-true
    w280 = T2 0 items=["PercentOutput"=0, "Position"=1, "Velocity"=2, "Current"=3, "Follower"=5, "MotionProfile"=6, "MotionMagic"=7, "MotionProfileArc"=10, "Disabled"=15] ("Control Mode")
    w287 = T2 0 items=["PercentOutput"=0, "Position"=1, "Velocity"=2, "Current"=3, "Follower"=5, "MotionProfile"=6, "MotionMagic"=7, "MotionProfileArc"=10, "Disabled"=15] ("Control Mode")
    # "blep"
    # "Conveyor Code"
    n228 = global read "Robot Global Data.vi" "horizontalConveyorMotorToggle"() -> (w283:bool)
    n229 = call "Read Sensors.vi"() -> ()  [unwired: 12 in]
    n230 = global read "Robot Global Data.vi" "killSwitch"() -> (w277:bool)
    n231 = global read "Robot Global Data.vi" "verticalConveyorDown"() -> (w286:bool)
    n232 = global read "Robot Global Data.vi" "verticalConveyorUp"() -> (w290:bool)
    n233 = case shown="False" w283 {
      tunnel: [w318 w337] -> w279
      tunnel: w277 -> [w317 _]
      frame False {
        n234 = case shown="False" w317 {
          tunnel: [w319 0.0] -> w318
          frame False {
            n235 = global read "Robot Global Data.vi" "conveyorSensor03"() -> (w320:bool)
            n236 = case shown="False" w320 {
              tunnel: [w325 0.0] -> w319
              frame False {
                n237 = global read "Robot Global Data.vi" "conveyorSensor04"() -> (w323:bool)
                n238 = global read "Robot Global Data.vi" "conveyorSensor02"() -> (w324:bool)
                n239 = global read "Robot Global Data.vi" "conveyorSensor01"() -> (w322:bool)
                n240 = Not(x=w324) -> (.not. x?=w327:bool)
                n241 = Or(x=w323, y=w322) -> (x .or. y?=w321:bool)
                n242 = And(x=w321, y=w327) -> (x .and. y?=w326:bool)
                n243 = case shown="False" w326 {
                  tunnel: [w329 -0.5] -> w325
                  tunnel: w324 -> [w331 _]
                  tunnel: w321 -> [w328 _]
                  frame False {
                    n244 = And(x=w328, y=w331) -> (x .and. y?=w330:bool)
                    n245 = case shown="False" w330 {
                      tunnel: [0.0 -0.5] -> w329
                      frame False {
                      }
                      frame True {
                      }
                    }
                  }
                  frame True {
                  }
                }
              }
              frame True {
              }
            }
          }
          frame True {
          }
        }
      }
      frame True {
        n246 = Negate(x=0.5) -> (-x=w337:dbl)
      }
    }
    n247 = case shown="False" w290 {
      tunnel: [w292 w315] -> w285
      tunnel: w286 -> [w293 _]
      tunnel: w277 -> [w291 _]
      frame False {
        n248 = case shown="False" w293 {
          tunnel: [w295 0.6] -> w292
          tunnel: w291 -> [w294 _]
          frame False {
            n249 = case shown="False" w294 {
              tunnel: [w296 0.0] -> w295
              frame False {
                n250 = global read "Robot Global Data.vi" "conveyorSensor03"() -> (w297:bool)
                n251 = case shown="False" w297 {
                  tunnel: [w302 0.0] -> w296
                  frame False {
                    n252 = global read "Robot Global Data.vi" "conveyorSensor04"() -> (w300:bool)
                    n253 = global read "Robot Global Data.vi" "conveyorSensor02"() -> (w301:bool)
                    n254 = global read "Robot Global Data.vi" "conveyorSensor01"() -> (w299:bool)
                    n255 = Not(x=w301) -> (.not. x?=w304:bool)
                    n256 = Or(x=w300, y=w299) -> (x .or. y?=w298:bool)
                    n257 = And(x=w298, y=w304) -> (x .and. y?=w303:bool)
                    n258 = case shown="False" w303 {
                      tunnel: [w306 -0.6] -> w302
                      tunnel: w301 -> [w308 _]
                      tunnel: w298 -> [w305 _]
                      frame False {
                        n259 = And(x=w305, y=w308) -> (x .and. y?=w307:bool)
                        n260 = case shown="False" w307 {
                          tunnel: [0.0 -0.6] -> w306
                          frame False {
                          }
                          frame True {
                          }
                        }
                      }
                      frame True {
                      }
                    }
                  }
                  frame True {
                  }
                }
              }
              frame True {
              }
            }
          }
          frame True {
            (unwired) 0.0
          }
        }
      }
      frame True {
        (unwired) 0.0
        # "Vertical Conveyor Moving Up"
        n261 = Negate(x=0.6) -> (-x=w315:dbl)
      }
    }
    n262 = call <vilib>:"CTRE_Phoenix_MotorControl_RefNumRegistryGet.vi"("refnum name"="verticalConveyorMotor") -> ("PhoenixMotorControlDevRef"=w288:T3)  [unwired: 9 in, 1 out]
    n263 = call <vilib>:"CTRE_Phoenix_MotorControl_RefNumRegistryGet.vi"("refnum name"="horizontalConveyorMotor") -> ("PhoenixMotorControlDevRef"=w281:T3)  [unwired: 9 in, 1 out]
    n264 = Wait (ms)(milliseconds to wait=u32 50) -> ()  [unwired: 1 out]
    n265 = call <vilib>:"CTRE_Phoenix_MotorControl_Set.vi"("Output"=w285, "Control Mode"=w287, "PhoenixMotorControlDevRef"=w288) -> ()  [unwired: 7 in, 2 out]
    n266 = call <vilib>:"CTRE_Phoenix_MotorControl_Set.vi"("Output"=w279, "Control Mode"=w280, "PhoenixMotorControlDevRef"=w281) -> ()  [unwired: 7 in, 2 out]
  }
  n267 = while {
    stop <- FALSE stop-if-true
    n268 = global read "Robot Global Data.vi" "servoDown"() -> (w339:bool)
    n269 = global read "Robot Global Data.vi" "servoOut"() -> (w341:bool)
    n270 = global read "Robot Global Data.vi" "servoUp"() -> (w342:bool)
    n271 = case shown="True" w339 {
      frame False {
      }
      frame True {
        n272 = global write "Robot Global Data.vi" "servoAngle"(190.0 ("servoAngle")) -> ()
        n273 = global write "Robot Global Data.vi" "servoOut"(FALSE ("servoOut")) -> ()
        n274 = global write "Robot Global Data.vi" "servoUp"(FALSE ("servoOut")) -> ()
      }
    }
    n275 = case shown="True" w341 {
      frame False {
      }
      frame True {
        n276 = global write "Robot Global Data.vi" "servoAngle"(110.0 ("servoAngle")) -> ()
        n277 = global write "Robot Global Data.vi" "servoDown"(FALSE ("servoOut")) -> ()
        n278 = global write "Robot Global Data.vi" "servoUp"(FALSE ("servoOut")) -> ()
      }
    }
    n279 = case shown="True" w342 {
      frame False {
      }
      frame True {
        n280 = global write "Robot Global Data.vi" "servoAngle"(20.0 ("servoAngle")) -> ()
        n281 = global write "Robot Global Data.vi" "servoDown"(FALSE ("servoOut")) -> ()
        n282 = global write "Robot Global Data.vi" "servoOut"(FALSE ("servoOut")) -> ()
      }
    }
    n283 = global read "Robot Global Data.vi" "servoAngle"() -> (w343:dbl)
    n284 = call <vilib>:"WPI_ServoRefNum Registry Get.vi"("refnum name"="cameraServo") -> ("ServoDeviceRef"=w345:T14)  [unwired: 9 in, 1 out]
    n285 = call <vilib>:"WPI_ServoSetAngle.vi"("Angle"=w343, "ServoDeviceRef"=w345) -> ()  [unwired: 8 in, 2 out]
  }
  n286 = while {
    stop <- FALSE stop-if-true
    w375 = T2 0 items=["PercentOutput"=0, "Position"=1, "Velocity"=2, "Current"=3, "Follower"=5, "MotionProfile"=6, "MotionMagic"=7, "MotionProfileArc"=10, "Disabled"=15] ("Control Mode")
    # "make sure the output does not have negative speed"
    # "the reciperical of time pre count is count pre time which will givr us the current revs. per second"
    # "PID is giving us Acceleration"
    # "motor speed in %\nVELOCITY"
    n287 = global read "Robot Global Data.vi" "shooterEncoderWantedRps"() -> (w364:dbl)
    n288 = global read "Robot Global Data.vi" "shooterEncoderCurrentRps"() -> (w355:dbl)
    n289 = global read "Robot Global Data.vi" "shooter"() -> (w371:bool)
    n290 = call <vilib>:"WPI_CounterRefNum Registry Get.vi"("refnum name"="shooterEncoder") -> ("error out"=w366:errorcluster, "CounterDevRef"=w365:T15)  [unwired: 9 in]
    n291 = call <vilib>:"WPI_CounterGet.vi"("error in (no error)"=w366, "CounterDevRef in"=w365) -> ("Period (sec)"=w363:dbl)  [unwired: 4 in, 5 out]
    n292 = Select(t=145.0, s=w371, f=0.0) -> (s? t:f=w361:dbl)
    n293 = Reciprocal(x=w363) -> (1/x=w362:dbl)
    n294 = global write "Robot Global Data.vi" "shooterEncoderWantedRps"(w361) -> ()
    n295 = global write "Robot Global Data.vi" "shooterEncoderCurrentRps"(w362) -> ()
    n296 = call-poly <vilib>:"PID.vi"("output range"=cluster{"output high":dbl, "output low":dbl} {"output high"=1.0, "output low"=-1.0}, "PID gains"=T10 {"proportional gain (Kc)"=0.0003, "integral time (Ti, min)"=0.0, "derivative time (Td, min)"=0.0}, "process variable"=w355, "setpoint"=w364) -> ("output"=w372:dbl)  [unwired: 6 in, 1 out]
    n297 = global read "Robot Global Data.vi" "shooterPercentOutput"() -> (w373:dbl)
    n298 = Add(x=w373, y=w372) -> (x+y=w357:dbl)
    n299 = Less Or Equal To 0?(x=w357) -> (x <= 0?=w360:bool)
    n300 = global read "Robot Global Data.vi" "shooterPercentOutput"() -> (w368:dbl)
    n301 = Select(t=0.0, s=w360, f=w357) -> (s? t:f=w358:dbl)
    n302 = global write "Robot Global Data.vi" "shooterPercentOutput"(w358) -> ()
    n303 = call <vilib>:"CTRE_Phoenix_MotorControl_RefNumRegistryGet.vi"("refnum name"="shooterMotor02") -> ("PhoenixMotorControlDevRef"=w376:T3)  [unwired: 9 in, 1 out]
    n304 = Wait (ms)(milliseconds to wait=u32 50) -> ()  [unwired: 1 out]
    n305 = Negate(x=w368) -> (-x=w374:dbl)
    n306 = call <vilib>:"CTRE_Phoenix_MotorControl_RefNumRegistryGet.vi"("refnum name"="shooterMotor01") -> ("PhoenixMotorControlDevRef"=w378:T3)  [unwired: 9 in, 1 out]
    n307 = call-poly <vilib>:"NT Write Value.vi"("Numeric"=w355, "Name"="RPS") -> ()  [unwired: 9 in, 1 out]
    n308 = call <vilib>:"CTRE_Phoenix_MotorControl_Set.vi"("Output"=w374, "Control Mode"=w375, "PhoenixMotorControlDevRef"=w376) -> ()  [unwired: 7 in, 2 out]
    n309 = call <vilib>:"CTRE_Phoenix_MotorControl_Set.vi"("Output"=w374, "Control Mode"=w375, "PhoenixMotorControlDevRef"=w378) -> ()  [unwired: 7 in, 2 out]
  }
  n310 = while {
    stop <- FALSE stop-if-true
    w392 = T2 0 items=["PercentOutput"=0, "Position"=1, "Velocity"=2, "Current"=3, "Follower"=5, "MotionProfile"=6, "MotionMagic"=7, "MotionProfileArc"=10, "Disabled"=15] ("Control Mode")
    # "no pid stuff \njust set motor outputs"
    # "math"
    # "current encoder * [( range of degrees) / (\"max out\" - \"max in')]\n= current degrees"
    # "enc. value at \"max in\""
    # "enc. value at \"max out\""
    # "This converts current encoder count to actual angles."
    # "SHOOTER ANGLE MOTOR"
    # "range of degrees"
    n311 = global read "Robot Global Data.vi" "manualShooterAngleDown"() -> (w396:bool)
    n312 = global read "Robot Global Data.vi" "manualShooterAngleUp"() -> (w395:bool)
    n313 = global read "Robot Global Data.vi" "shooterMotorStartValue"() -> (w397:dbl)
    n314 = call <vilib>:"CTRE_Phoenix_MotorControl_RefNumRegistryGet.vi"("refnum name"="shooterAngleMotor") -> ("error out"=w399:errorcluster, "PhoenixMotorControlDevRef"=w400:T3)  [unwired: 9 in]
    n315 = call-poly <vilib>:"CTRE_Phoenix_MotorController_Get_Enhanced.vi"("PhoenixMotorControlDevRef"=w400, "error in"=w399) -> ("Quadrature Position"=w398:i32)  [unwired: 10 in, 3 out]
    n316 = disable-structure shown="Enabled" {
      disable-tunnel: w396 -> [w406 w459]
      disable-tunnel: w395 -> [w405 w462]
      disable-tunnel: [w404 w458] -> w393
      frame Disabled {
        n317 = case shown="False" w405 {
          tunnel: w406 -> [w408 _]
          tunnel: [w407 w449] -> w404
          frame False {
            # "Upper POV not being pressed"
            n318 = case shown="False" w408 {
              tunnel: [w409 w441] -> w407
              frame False {
                # "enc. val at\n\"max in\"\ndeg IRL"
                # "Checks if any of the presets are being pressed, then set those desired angles. \nThe PID code that sets the output is put into here too."
                n319 = global read "Robot Global Data.vi" "shooterAnglePreset01"() -> (w410:bool)
                n320 = global read "Robot Global Data.vi" "shooterAnglePreset03"() -> (w413:bool)
                n321 = global read "Robot Global Data.vi" "shooterAnglePreset04"() -> (w412:bool)
                n322 = disable-structure shown="Enabled" {
                  disable-tunnel: [w417 w424] -> w409
                  frame Enabled {
                    # "We need to adjust the PID values to match \nthe bot."
                    n323 = global read "Robot Global Data.vi" "shooterMotorWantedAngle"() -> (w416:dbl)
                    n324 = global read "Robot Global Data.vi" "shooterMotorActualAngle"() -> (w415:dbl)
                    n325 = call-poly <vilib>:"PID.vi"("output range"=cluster{"output high":dbl, "output low":dbl} {"output high"=0.25, "output low"=-0.25}, "PID gains"=T10 {"proportional gain (Kc)"=0.0002, "integral time (Ti, min)"=0.0, "derivative time (Td, min)"=0.0}, "process variable"=w415, "setpoint"=w416) -> ("output"=w417:dbl)  [unwired: 6 in, 1 out]
                  }
                  frame Disabled {
                    # "spin in the corrent direction"
                    # "accepted error range of wanted angle\nand current angle"
                    n326 = global read "Robot Global Data.vi" "shooterMotorWantedAngle"() -> (w430:dbl)
                    n327 = global read "Robot Global Data.vi" "shooterMotorActualAngle"() -> (w429:dbl)
                    n328 = Subtract(x=w430, y=w429) -> (x-y=w421:dbl)
                    n329 = Greater Than 0?(x=w421) -> (x > 0?=w422:bool)
                    n330 = In Range and Coerce(upper limit=0.5, x=w421, lower limit=-0.5) -> (In Range?=w426:bool)  [unwired: 1 out]
                    n331 = Select(t=-0.25, s=w422, f=0.25) -> (s? t:f=w423:dbl)
                    n332 = Select(t=0.0, s=w426, f=w423) -> (s? t:f=w424:dbl)
                  }
                }
                n333 = case shown="False" w410 {
                  tunnel: w413 -> [w433 _]
                  tunnel: w412 -> [w432 _]
                  tunnel: [w431 0.0] -> w411
                  frame False {
                    n334 = case shown="False" w433 {
                      tunnel: w432 -> [w435 _]
                      tunnel: [w434 11.34] -> w431
                      frame False {
                        n335 = case shown="False" w435 {
                          tunnel: [w436 9.85] -> w434
                          frame False {
                            n336 = global read "Robot Global Data.vi" "shooterMotorWantedAngle"() -> (w436:dbl)
                          }
                          frame True {
                            # "behind wheel"
                          }
                        }
                      }
                      frame True {
                        # "end of trench preset"
                      }
                    }
                  }
                  frame True {
                    # "init line"
                  }
                }
                n337 = global write "Robot Global Data.vi" "shooterMotorWantedAngle"(w411) -> ()
              }
              frame True {
                # "Lower POV being pressed. Manual control."
                n338 = global read "Robot Global Data.vi" "shooterAngleOverride"() -> (w440:bool)
                n339 = case shown="False" w440 {
                  tunnel: [w444 0.25 ("Output")] -> w441
                  frame False {
                    n340 = global read "Robot Global Data.vi" "shooterMotorActualAngle"() -> (w443:dbl)
                    n341 = Less Or Equal To 0?(x=w443) -> (x <= 0?=w442:bool)
                    n342 = case shown="False" w442 {
                      tunnel: [0.25 ("Output") 0.0 ("Output")] -> w444
                      frame False {
                      }
                      frame True {
                      }
                    }
                  }
                  frame True {
                  }
                }
              }
            }
          }
          frame True {
            # "Upper POV being pressed. Manual Control of shooter angle motor."
            n343 = global read "Robot Global Data.vi" "shooterAngleOverride"() -> (w448:bool)
            n344 = case shown="False" w448 {
              tunnel: [w454 0.25 ("Output")] -> w450
              frame False {
                n345 = global read "Robot Global Data.vi" "shooterMotorActualAngle"() -> (w453:dbl)
                n346 = Greater Or Equal?(x=w453, y=32.0) -> (x >= y?=w451:bool)
                n347 = case shown="True" w451 {
                  tunnel: [0.25 ("Output") 0.0] -> w454
                  frame False {
                  }
                  frame True {
                  }
                }
              }
              frame True {
              }
            }
            n348 = Negate(x=w450) -> (-x=w449:dbl)
          }
        }
      }
      frame Enabled {
        w461 = 0.5  # Wanted angle rate of change
        # "We need to adjust the PID values to match \nthe bot."
        n349 = global read "Robot Global Data.vi" "shooterMotorWantedAngle"() -> (w466:dbl)
        n350 = global read "Robot Global Data.vi" "shooterMotorActualAngle"() -> (w467:dbl)
        n351 = case shown="False" w462 {
          tunnel: w461 -> [w469 w497]
          tunnel: [w468 w496] -> w460
          tunnel: w459 -> [w470 _]
          frame False {
            n352 = case shown="False" w470 {
              tunnel: w469 -> [_ w488]
              tunnel: [w471 w484] -> w468
              frame False {
                n353 = global read "Robot Global Data.vi" "shooterAnglePreset01"() -> (w472:bool)
                n354 = global read "Robot Global Data.vi" "shooterAnglePreset03"() -> (w474:bool)
                n355 = global read "Robot Global Data.vi" "shooterAnglePreset04"() -> (w473:bool)
                n356 = case shown="False" w472 {
                  tunnel: w474 -> [w477 _]
                  tunnel: w473 -> [w476 _]
                  tunnel: [w475 17.0] -> w471
                  frame False {
                    n357 = case shown="False" w477 {
                      tunnel: w476 -> [w479 _]
                      tunnel: [w478 21.0] -> w475
                      frame False {
                        n358 = case shown="False" w479 {
                          tunnel: [w480 26.85] -> w478
                          frame False {
                            n359 = global read "Robot Global Data.vi" "shooterMotorWantedAngle"() -> (w480:dbl)
                          }
                          frame True {
                            # "behind wheel"
                          }
                        }
                      }
                      frame True {
                        # "end of trench preset"
                      }
                    }
                  }
                  frame True {
                    # "init line"
                  }
                }
              }
              frame True {
                # "31 not 38 cuz squishy"
                n360 = global read "Robot Global Data.vi" "shooterMotorWantedAngle"() -> (w487:dbl)
                n361 = global read "Robot Global Data.vi" "shooterAngleOverride"() -> (w486:bool)
                n362 = Subtract(x=w487, y=w488) -> (x-y=w485:dbl)
                n363 = case shown="False" w486 {
                  tunnel: w485 -> [w492 w493]
                  tunnel: [w489 w493] -> w484
                  frame False {
                    n364 = In Range and Coerce(upper limit=31.0, x=w492, lower limit=0.0) -> (coerced(x)=w489:dbl)  [unwired: 1 out]
                  }
                  frame True {
                  }
                }
              }
            }
          }
          frame True {
            n365 = global read "Robot Global Data.vi" "shooterMotorWantedAngle"() -> (w498:dbl)
            n366 = global read "Robot Global Data.vi" "shooterAngleOverride"() -> (w494:bool)
            n367 = Add(x=w497, y=w498) -> (x+y=w495:dbl)
            n368 = case shown="False" w494 {
              tunnel: [w499 w503] -> w496
              tunnel: w495 -> [w502 w503]
              frame False {
                n369 = In Range and Coerce(upper limit=31.0, x=w502, lower limit=0.0) -> (coerced(x)=w499:dbl)  [unwired: 1 out]
              }
              frame True {
              }
            }
          }
        }
        n370 = call-poly <vilib>:"PID.vi"("output range"=cluster{"output high":dbl, "output low":dbl} {"output high"=0.25, "output low"=-0.25}, "PID gains"=T10 {"proportional gain (Kc)"=0.089, "integral time (Ti, min)"=0.0, "derivative time (Td, min)"=0.0}, "process variable"=w467, "setpoint"=w466) -> ("output"=w463:dbl)  [unwired: 6 in, 1 out]
        n371 = Negate(x=w463) -> (-x=w458:dbl)
        n372 = global write "Robot Global Data.vi" "shooterMotorWantedAngle"(w460) -> ()
      }
    }
    n373 = Subtract(x=w398, y=w397) -> (x-y=w390:dbl)
    n374 = Multiply(x=38.0, y=w390) -> (x*y=w386:dbl)
    n375 = Subtract(x=-1112.0, y=6237.0) -> (x-y=w385:dbl)
    n376 = Divide(x=w386, y=w385) -> (x/y=w384:dbl)
    n377 = global write "Robot Global Data.vi" "shooterMotorActualAngle"(w384) -> ()
    n378 = call <vilib>:"CTRE_Phoenix_MotorControl_RefNumRegistryGet.vi"("refnum name"="shooterAngleMotor") -> ("PhoenixMotorControlDevRef"=w394:T3)  [unwired: 9 in, 1 out]
    n379 = Wait (ms)(milliseconds to wait=u32 50) -> ()  [unwired: 1 out]
    n380 = call <vilib>:"CTRE_Phoenix_MotorControl_Set.vi"("Output"=w393, "Control Mode"=w392, "PhoenixMotorControlDevRef"=w394) -> ()  [unwired: 7 in, 2 out]
  }
